vi "Create.vi"(8 "error in (no error)":errorcluster, 10 "Result":refnum<class "Result.lvclass">) -> (0 "error out":errorcluster, 3 "Future out":refnum<class "Future.lvclass">)   [LabVIEW 2017, in "Futures.lvlib" / "Future.lvclass"]
uses:
  Future.lvclass
  Result/Result.lvclass
  Future.lvclass/Future.ctl
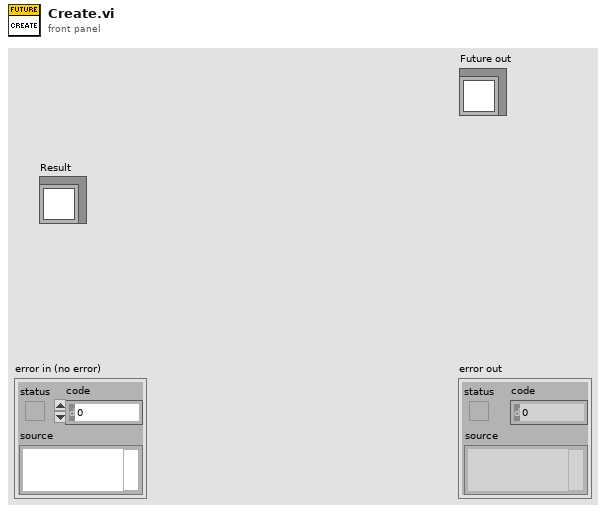
[diagram p1: front panel]
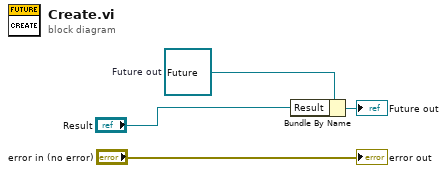
[diagram p0: block diagram]
diagram:
  w4 = refnum<class "Future.lvclass"> refnum  # Future out
  n1 = Bundle By Name(cluster=w4, "Result"="Result") -> (→"Future out":refnum<class "Future.lvclass">)
  "error out" <- "error in (no error)"
